vi "DrawLine.vi"(1 "Color":u32(colorbox)=16711680, 2 "Edge Points":T2, 3 "img in":T1) -> (0 "Image Out":T1)   [LabVIEW 2014]
uses:
  <vilib>/vision/Image Controls.llb/IMAQ Image.ctl
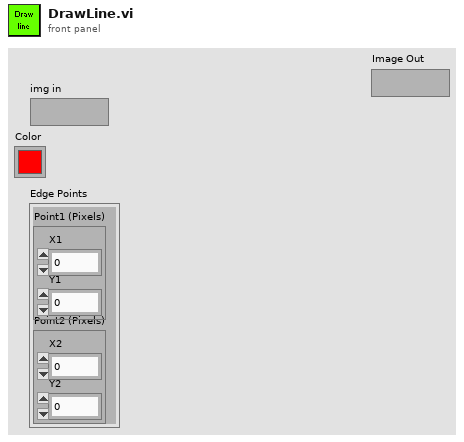
[diagram p1: front panel]
types:
  T1 = typedef "IMAQ Image.ctl" = refnum<image>
  T2 = cluster{"Point1 (Pixels)":cluster{"X1":sgl, "Y1":sgl}, "Point2 (Pixels)":cluster{"X2":sgl, "Y2":sgl}}
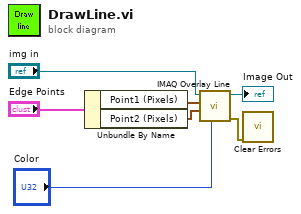
[diagram p0: block diagram]
diagram:
  n1 = Unbundle By Name("Edge Points") -> ("Point1 (Pixels)"=w5:cluster{"X1":sgl, "Y1":sgl}, "Point2 (Pixels)"=w6:cluster{"X2":sgl, "Y2":sgl})
  n2 = call "IMAQ Overlay Line"("Color"="Color", "End Point"=w6, "Start Point"=w5, "Image"="img in") -> ("error out"=w1:errorcluster, "Image Out"=→"Image Out":T1)  [unwired: 6 in]
  n3 = call <vilib>:"Clear Errors.vi"("error in (no error)"=w1) -> ()  [unwired: 5 in, 2 out]
